vi "Set Theme Data.vi"(7 "VI Refnum":refnum<vi>, 8 "error in":errorcluster, 10 "Theme":u16(ring)=3 items=["Light Theme", "Light Medium Contrast", "Light High Contrast", "Dark Theme", "Dark Medium Contrast", "Dark High Constrast"], 11 "Material Theme.lvclass":refnum<class "Material Theme.lvclass">) -> (0 "error out":errorcluster)   [LabVIEW 2021, in "TSC Material Theme.lvlib" / "Material Theme.lvclass"]
doc: "Set the VI's User Tag data to track the theme and theme mode applied.\n\n<b>Code Developed By:</b> +\nDaniel Coons +\nTechnology Service Corporation +\nwww.tsc.com/atcs"
uses:
  Material Theme.lvclass
  Material Theme.lvclass/Material Theme.ctl
  <vilib>/UserTags/UserTags.lvlib
  Material SubVIs/Material SubVIs.lvlib
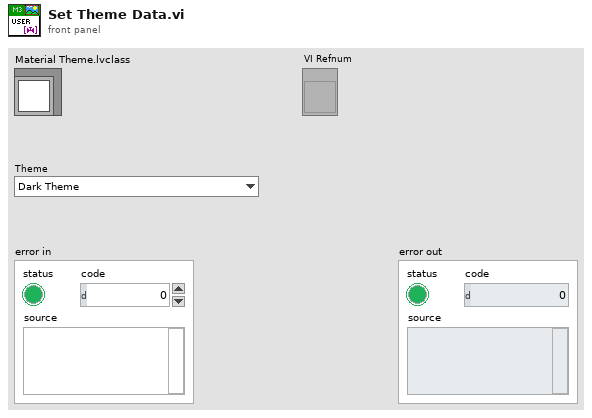
[diagram p1: front panel]
types:
  T1 = typedef "AB_Relative_Path_Type.ctl" = enum16{"<none>", "relativeToCommon", "relativeToAppDir", "relativeToProject"}
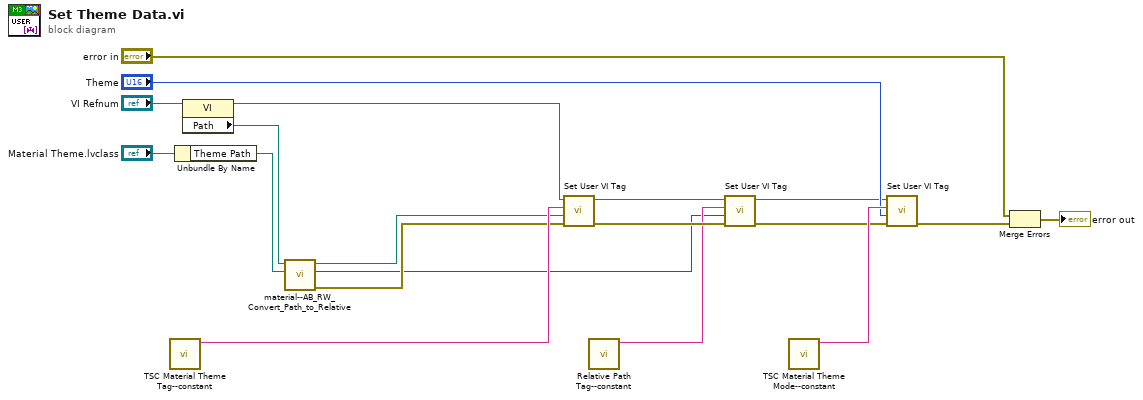
[diagram p0: block diagram]
diagram:
  n1 = call "TSC Material Theme Tag--constant.vi"() -> ("Theme Path Tag"=w16:string)  [unwired: 11 in]
  n2 = Unbundle By Name("Material Theme.lvclass") -> ("Theme Path"=w10:path)
  n3 = property class="VI"(reference="VI Refnum") -> (reference out=w9:refnum<vi>, "Path"=w8:path)  [unwired: 1 in, 1 out]
  n4 = call "material--AB_RW_Convert_Path_to_Relative.vi"("Theme Path"=w10, "VI Path"=w8) -> ("error out"=w2:errorcluster, "relativeType"=w1:T1, "newPath"=w7:path)  [unwired: 7 in]
  n5 = call <vilib>:"Set User VI Tag.vi"("error in (no error)"=w2, "Value"=w7, "Tag Name"=w16, "VI Refnum"=w9) -> ("error out"=w19:errorcluster, "dup VI Refnum"=w5:refnum<vi>)  [unwired: 5 in, 1 out]
  n6 = call "Relative Path Tag--constant.vi"() -> ("Relative Path Tag"=w3:string)  [unwired: 11 in]
  n7 = call <vilib>:"Set User VI Tag.vi"("error in (no error)"=w19, "Value"=w1, "Tag Name"=w3, "VI Refnum"=w5) -> ("error out"=w6:errorcluster, "dup VI Refnum"=w4:refnum<vi>)  [unwired: 5 in, 1 out]
  n8 = call "TSC Material Theme Mode--constant.vi"() -> ("Theme Path Tag"=w14:string)  [unwired: 11 in]
  n9 = call <vilib>:"Set User VI Tag.vi"("error in (no error)"=w6, "Value"="Theme", "Tag Name"=w14, "VI Refnum"=w4) -> ("error out"=w18:errorcluster)  [unwired: 5 in, 2 out]
  n10 = Merge Errors("error in", w18) -> (→"error out":errorcluster)
